vi "Load UserPrefs.vi"(8 "error in (no error)":errorcluster, 11 "BluelinesRedlines in":refnum<class "BluelinesRedlines.lvclass">) -> (0 "error out":errorcluster, 3 "BluelinesRedlines out":refnum<class "BluelinesRedlines.lvclass">)   [LabVIEW 2020, in "VolatusGUIElements.lvlib" / "BluelinesRedlines.lvclass"]
uses:
  BluelinesRedlines.lvclass
  VolatusGUI/BluelinesRedlines Source/BLRL Type.ctl
  BluelinesRedlines.lvclass/BluelinesRedlines.ctl
  User BluelinesRedlines/User BluelinesRedlines.lvclass
  C:/dev/lv20CE/relink/lv-volatus/VolatusGUI/BluelinesRedlines Source/BluelinesRedlines Source.lvclass
  lv-userprefs/User Prefs/Pref Group/Pref Group.lvclass
  VolatusGUI/BluelinesRedlines Source/BluelinesRedlines Source.lvclass
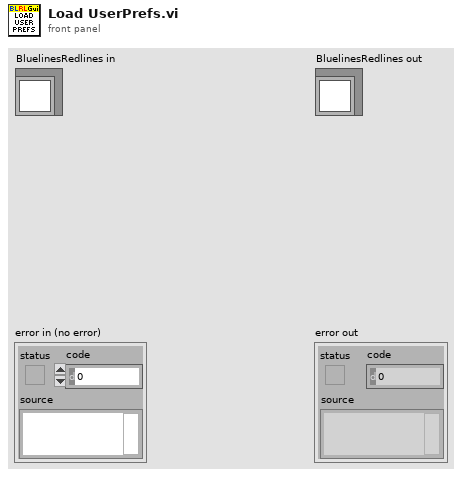
[diagram p1: front panel]
types:
  T1 = typedef "VolatusGUI.lvlib/BluelinesRedlines Source.lvclass/BLRL Type.ctl" = enum16{"Blueline", "Redline"}
  T2 = map{string, refnum<class "BluelinesRedlines Source.lvclass">}
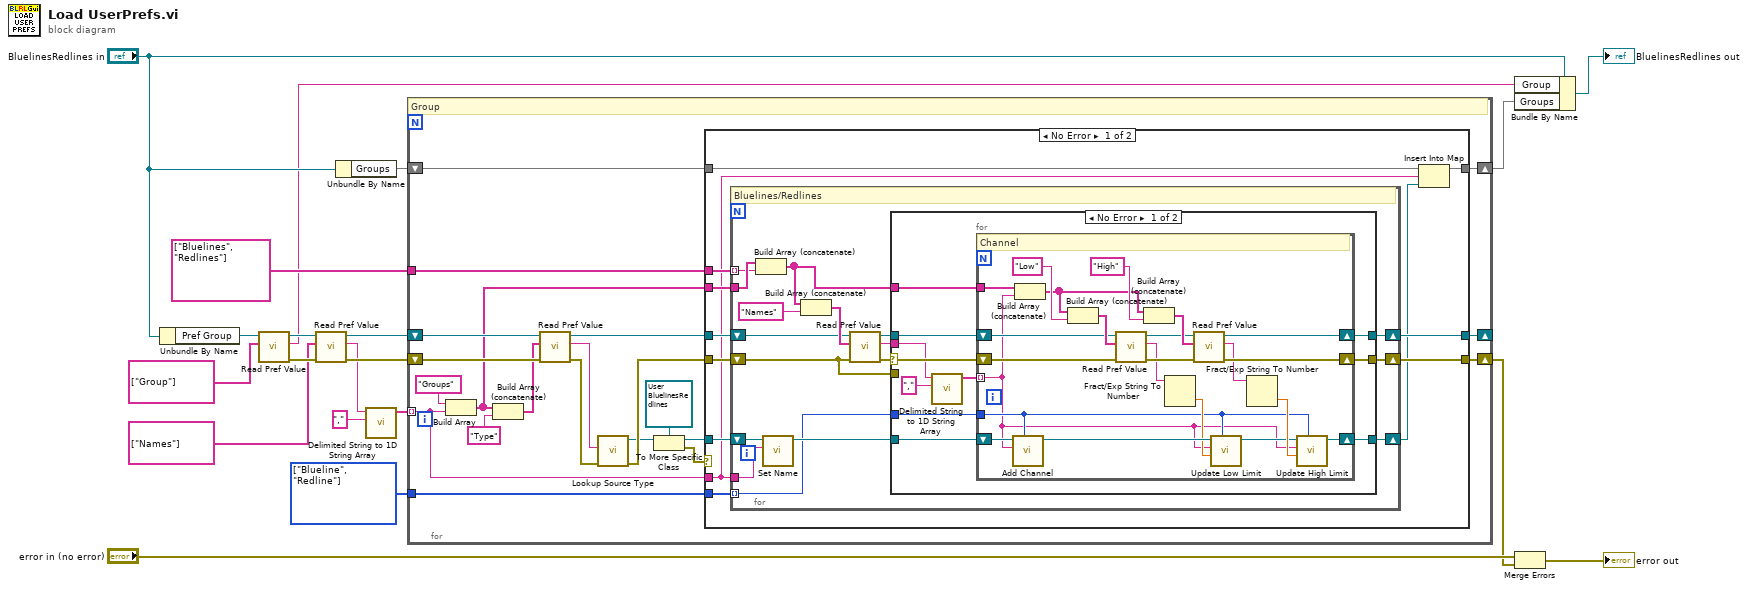
[diagram p0: block diagram]
diagram:
  w9 = T1[] [enum."Blueline", enum."Redline"] items=["Blueline", "Redline"]
  n1 = Unbundle By Name("BluelinesRedlines in") -> ("Pref Group"=w18:refnum<class "Pref Group.lvclass">)
  n2 = call "Read Pref Value.vi"("Pref Hierarchy"=string[] ["Group"], "Pref Group in"=w18) -> ("error out"=w15:errorcluster, "Value"=w3:string, "Pref Group out"=w16:refnum<class "Pref Group.lvclass">)  [unwired: 7 in]
  n3 = call "Read Pref Value.vi"("error in (no error)"=w15, "Pref Hierarchy"=string[] ["Names"], "Pref Group in"=w16) -> ("error out"=w20:errorcluster, "Value"=w13:string, "Pref Group out"=w10:refnum<class "Pref Group.lvclass">)  [unwired: 6 in]
  n4 = Unbundle By Name("BluelinesRedlines in") -> ("Groups"=w6:T2)
  n5 = call <vilib>:"Delimited String to 1D String Array.vi"("delimiter"=",", "delimited string"=w13) -> ("string array"=w11:string[])  [unwired: 9 in]
  n6 = for {
    tunnel: w11 -> [w27] mode=indexing
    shift-right: [w23] -> w1
    shift-left: w20 -> [w37]
    shift-right: [w24] -> _
    shift-left: w10 -> [w38]
    tunnel: w9 -> [w26]
    tunnel: string[] ["Bluelines", "Redlines"] -> [w25]
    shift-right: [w21] -> w4
    shift-left: w6 -> [w22]
    # "Group"
    n7 = Build Array("Groups" ("String"), w27) -> (w28:string[])
    n8 = Build Array (concatenate)(w28, "Type" ("String")) -> (w36:string[])
    n9 = call "Read Pref Value.vi"("error in (no error)"=w37, "Pref Hierarchy"=w36, "Pref Group in"=w38) -> ("error out"=w34:errorcluster, "Value"=w35:string, "Pref Group out"=w29:refnum<class "Pref Group.lvclass">)  [unwired: 6 in]
    n10 = call "Lookup Source Type.vi"("error in (no error)"=w34, "Source Type"=w35) -> ("error out"=w41:errorcluster, "Source"=w33:refnum<class "BluelinesRedlines Source.lvclass">)  [unwired: 8 in]
    n11 = To More Specific Class(target class=refnum<class "User BluelinesRedlines.lvclass"> refnum ("VolatusGUIElements.lvlib:User BluelinesRedlines.lvclass"), reference=w33) -> (specific class reference=w31:refnum<class "User BluelinesRedlines.lvclass">, error out=w30:errorcluster)  [unwired: 1 in]
    n12 = case shown="No Error" w30 {
      tunnel: w31 -> [w53 _]
      tunnel: w29 -> [w50 w108]
      tunnel: w41 -> [w49 w109]
      tunnel: w28 -> [w52 _]
      tunnel: w27 -> [w43 _]
      tunnel: w26 -> [w51 _]
      tunnel: w25 -> [w48 _]
      tunnel: [w47 w108] -> w24
      tunnel: [w46 w109] -> w23
      tunnel: w22 -> [w45 w107]
      tunnel: [w44 w107] -> w21
      frame No Error {
        n13 = for {
          tunnel: w52 -> [w65]
          tunnel: w43 -> [w66]
          shift-right: [w55] -> w42
          shift-left: w53 -> [w68]
          tunnel: w51 -> [w60] mode=indexing
          shift-right: [w56] -> w47
          shift-left: w50 -> [w61]
          shift-right: [w57] -> w46
          shift-left: w49 -> [w58]
          tunnel: w48 -> [w64] mode=indexing
          # "Bluelines/Redlines"
          n14 = Build Array (concatenate)(w65, w64) -> (w54:string[])
          n15 = call "Set Name.vi"("Name"=w66, "User BluelinesRedlines in"=w68) -> ("User BluelinesRedlines out"=w67:refnum<class "User BluelinesRedlines.lvclass">)  [unwired: 8 in, 1 out]
          n16 = Build Array (concatenate)(w54, "Names" ("String")) -> (w62:string[])
          n17 = call "Read Pref Value.vi"("error in (no error)"=w58, "Pref Hierarchy"=w62, "Pref Group in"=w61) -> ("error out"=w59:errorcluster, "Value"=w70:string, "Pref Group out"=w69:refnum<class "Pref Group.lvclass">)  [unwired: 6 in]
          n18 = case shown="No Error" w59 {
            selector: w59 -> [w81 _]
            tunnel: w70 -> [w79 _]
            tunnel: w69 -> [w77 w105]
            tunnel: w67 -> [w76 w104]
            tunnel: w60 -> [w75 _]
            tunnel: w58 -> [_ w106]
            tunnel: [w72 w106] -> w57
            tunnel: [w71 w105] -> w56
            tunnel: [w73 w104] -> w55
            tunnel: w54 -> [w74 _]
            frame No Error {
              n19 = call <vilib>:"Delimited String to 1D String Array.vi"("delimiter"=",", "delimited string"=w79) -> ("string array"=w78:string[])  [unwired: 9 in]
              n20 = for {
                tunnel: w78 -> [w84] mode=indexing
                shift-right: [w82] -> w71
                shift-left: w77 -> [w95]
                shift-right: [w103] -> w72
                shift-left: w81 -> [w102]
                shift-right: [w83] -> w73
                shift-left: w76 -> [w98]
                tunnel: w75 -> [w85]
                tunnel: w74 -> [w97]
                # "Channel"
                n21 = call "Add Channel.vi"("Type"=w85, "Channel Name"=w84, "User BluelinesRedlines in"=w98) -> ("User BluelinesRedlines out"=w89:refnum<class "User BluelinesRedlines.lvclass">)  [unwired: 7 in, 1 out]
                n22 = Build Array (concatenate)(w97, w84) -> (w99:string[])
                n23 = Build Array (concatenate)(w99, "Low") -> (w96:string[])
                n24 = call "Read Pref Value.vi"("error in (no error)"=w102, "Pref Hierarchy"=w96, "Pref Group in"=w95) -> ("error out"=w92:errorcluster, "Value"=w91:string, "Pref Group out"=w93:refnum<class "Pref Group.lvclass">)  [unwired: 6 in]
                n25 = Build Array (concatenate)(w99, "High") -> (w94:string[])
                n26 = Fract/Exp String To Number(string=w91) -> (number=w88:dbl)  [unwired: 3 in, 1 out]
                n27 = call "Read Pref Value.vi"("error in (no error)"=w92, "Pref Hierarchy"=w94, "Pref Group in"=w93) -> ("error out"=w103:errorcluster, "Value"=w90:string, "Pref Group out"=w82:refnum<class "Pref Group.lvclass">)  [unwired: 6 in]
                n28 = call "Update Low Limit.vi"("Type"=w85, "Low Limit"=w88, "Channel Name"=w84, "User BluelinesRedlines in"=w89) -> ("User BluelinesRedlines out"=w86:refnum<class "User BluelinesRedlines.lvclass">)  [unwired: 6 in, 1 out]
                n29 = Fract/Exp String To Number(string=w90) -> (number=w87:dbl)  [unwired: 3 in, 1 out]
                n30 = call "Update High Limit.vi"("Type"=w85, "High Limit"=w87, "Channel Name"=w84, "User BluelinesRedlines in"=w86) -> ("User BluelinesRedlines out"=w83:refnum<class "User BluelinesRedlines.lvclass">)  [unwired: 6 in, 1 out]
              }
            }
            frame Error {
              # "Groups don't require a Bluelines or Redlines section to be defined."
            }
          }
        }
        n31 = Insert Into Map(map in=w45, key=w43, value=w42) -> (map out=w44:T2)  [unwired: 2 out]
      }
      frame Error {
        # "Only support User source for now but have factory pattern in place to be ready for future extension if needed."
      }
    }
  }
  n32 = Bundle By Name(cluster="BluelinesRedlines in", "Group"=w3, "Groups"=w4) -> (→"BluelinesRedlines out":refnum<class "BluelinesRedlines.lvclass">)
  n33 = Merge Errors("error in (no error)", w1) -> (→"error out":errorcluster)
